vi "getValue.vi"(8 "error in (no error)":errorcluster, 11 "IBoolean in":refnum<class "IBoolean.lvclass">) -> (0 "error out":errorcluster, 2 "Value out":bool, 3 "IBoolean out":refnum<class "IBoolean.lvclass">)   [LabVIEW 2022 SP3, in "openDAQ.lvlib" / "daqCoreTypes.lvlib" / "IBoolean.lvclass"]
uses:
  <instrlib>/openDAQ/Public/Classes/daqCoreTypes/IBoolean/IBoolean.lvclass
  C:/Program Files (x86)/National Instruments/LabVIEW 2022/instr.lib/openDAQ/Public/Classes/IBaseObject/IBaseObject.lvclass
  <instrlib>/openDAQ/Public/Classes/IBaseObject/IBaseObject.lvclass/IBaseObject.ctl
  <instrlib>/openDAQ/Public/Classes/IBaseObject/Accessor/Read reference.vi
  <instrlib>/openDAQ/Binaries/Windows/x86/copendaq32.dll
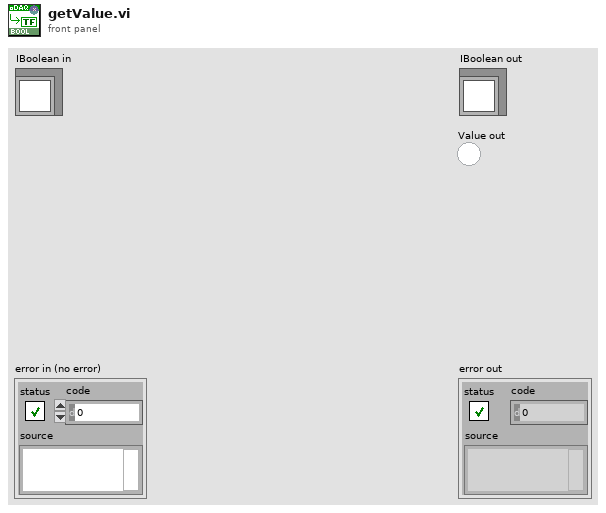
[diagram p1: front panel]
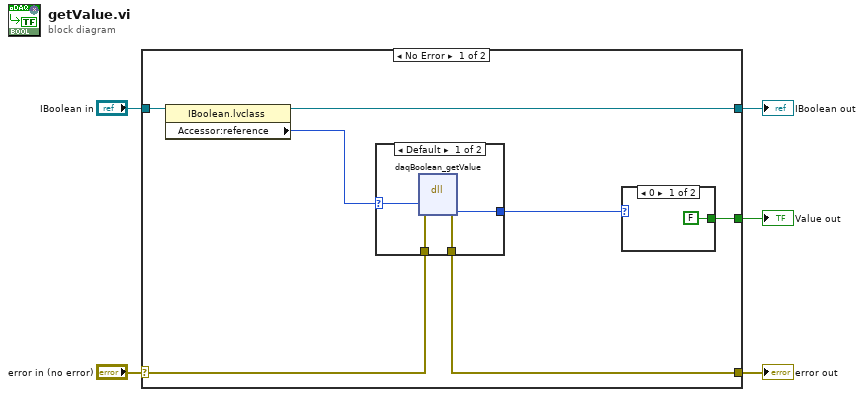
[diagram p0: block diagram]
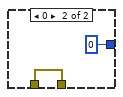
[diagram p2: hidden frame]
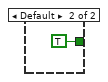
[diagram p3: hidden frame]
diagram:
  n1 = case shown="No Error" "error in (no error)" {
    selector: "error in (no error)" -> [w12 w22]
    tunnel: [w11 w22] -> w4
    tunnel: [w9 w21] -> w2
    tunnel: "IBoolean in" -> [w10 w21]
    tunnel: [w7 _] -> w1
    frame No Error {
      n2 = property class="IBoolean.lvclass"(reference=w10) -> (reference out=w9:refnum<class "IBoolean.lvclass">, "Accessor:reference"=w6:i64)  [unwired: 1 in, 1 out]
      n3 = case shown="Default" w6 {
        selector: w6 -> [w13 _]
        tunnel: w12 -> [w16 w18]
        tunnel: [w15 w18] -> w11
        tunnel: [w14 i64 0 ("value")] -> w8
        frame Default {
          n4 = dll-call lib="C:/Program Files (x86)/National Instruments/LabVIEW 2022/instr.lib/openDAQ/Binaries/Windows/x86/copendaq*.*" fn="daqBoolean_getValue"(error in=w16, "obj"=w13) -> (error out=w15:errorcluster, "value"=w14:i64)  [unwired: 5 in, 1 out]
        }
        frame 0 {
        }
      }
      n5 = case shown="0" w8 {
        tunnel: [FALSE TRUE] -> w7
        frame 0 {
        }
        frame Default {
        }
      }
    }
    frame Error {
    }
  }
  "error out" <- w4
  "IBoolean out" <- w2
  "Value out" <- w1
